vi "Error Processor.vi"(8 "error in (no error)":errorcluster, 11 "TCP Writer in":refnum<class "TCP Writer.lvclass">) -> (0 "error out":errorcluster, 3 "TCP Writer out":refnum<class "TCP Writer.lvclass">)   [LabVIEW 2026, in "TALOS.lvlib" / "TCP Writer.lvlib" / "TCP Writer.lvclass"]
doc: "Use this VI to process all the error that are solvable inside this specific uService. Whatever is not possible to process, let it leave this VI and it will be processed by the Error Manager of the Distributed System."
uses:
  TCP Writer.lvclass
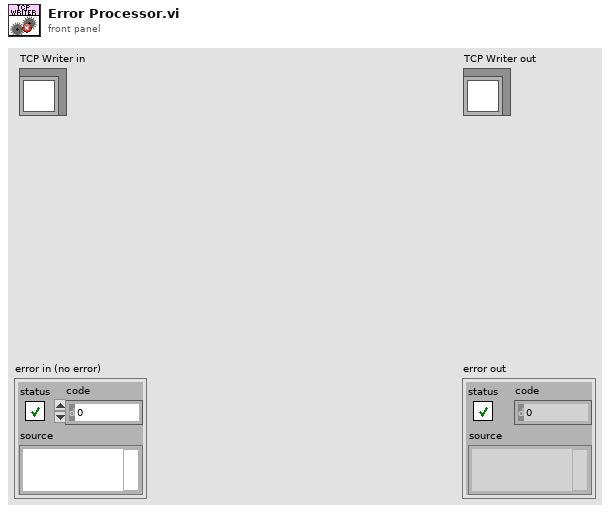
[diagram p1: front panel]
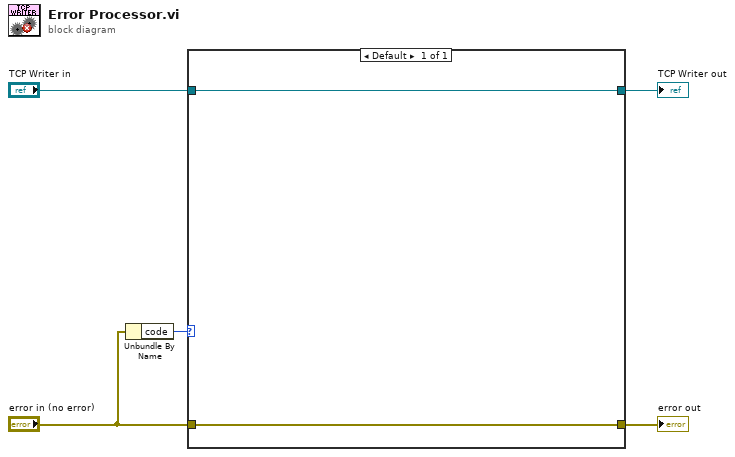
[diagram p0: block diagram]
diagram:
  n1 = Unbundle By Name("error in (no error)") -> ("code"=w1:i32)
  n2 = case shown="Default" w1 {
    tunnel: "error in (no error)" -> [w7]
    tunnel: [w7] -> w5
    tunnel: "TCP Writer in" -> [w6]
    tunnel: [w6] -> w4
    frame Default {
    }
  }
  "error out" <- w5
  "TCP Writer out" <- w4
